vi "Day1_boolean1.vi"() -> ()   [LabVIEW 2014]
panel:
  out "뒤집힌 배열":bool[](array[boolean])
  out "불리언 배열":bool[](array[boolean])
  in  "숫자형 2":u8 format="%.0b"
  in  "숫자형":u8 format="%.0b"
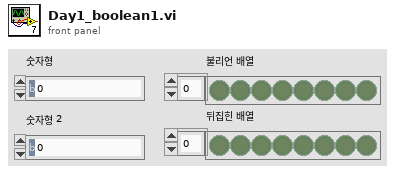
[diagram p1: front panel]
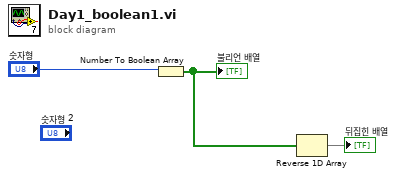
[diagram p0: block diagram]
diagram:
  n1 = Number To Boolean Array(number="숫자형") -> (Boolean array=w2:bool[])
  "불리언 배열" <- w2
  n2 = Reverse 1D Array(array=w2) -> (reversed array=→"뒤집힌 배열":bool[])
